vi "LVDimInterface.dis_remove_service.vi"(0 "my_serviceID":i32, 5 "error in (no error)":errorcluster) -> (19 "error out":errorcluster)   [LabVIEW 2015, in "LVDimInterface.lvlib"]
doc: "This routine can be called by the server program when a service stops beeing provided. \nThis routine will inform the Name server and all the clients using this service that it is no longer provided. The service can from then on be provided by another server.\n\nRemark: Please use a \"remove command' for removing command services\n\nHistory: 16-DEC-2005, Dietrich Beck\n\nCopyright (C)\nGesellschaft für Schwerionenforschung, GSI\nPlanckstr. 1\n64291 Darmstadt\nGermany\n\nContact: D.Beck@gsi.de \n\nThis program is free software; you can redistribute it and/or modify it under the terms of the \nGNU General Public License as published by the Free Software Foundation; either version 2 of the license, or (at your option) any later version.\n\nThis program is distributed in the hope that it will be useful, but WITHOUT ANY WARRANTY; without even the implied warranty of MERCHANTABILITY or FITNESS FOR A PARTICULAR PURPOSE. See the GNU General License for more details (http://www.gnu.org).\n\nGesellschaft für Schwerionenforschung, GSI\nPlanckstr. 1, 64291 Darmstadt, Germany\nFor all questions and ideas contact D. Beck.\nLast update: 16-DEC-2005"
uses:
  LVDimInterface.lvlib
  bin/libDimWrapper.dll
  bin/libDimWrapper.so
  bin/libDimWrapperSPL.dll
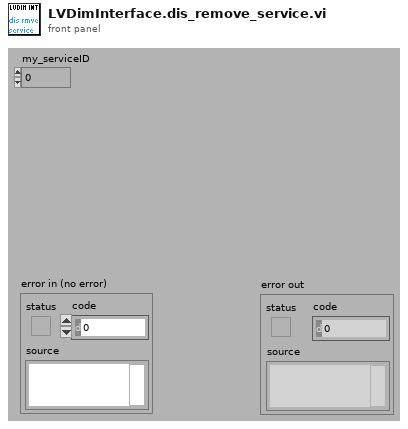
[diagram p1: front panel]
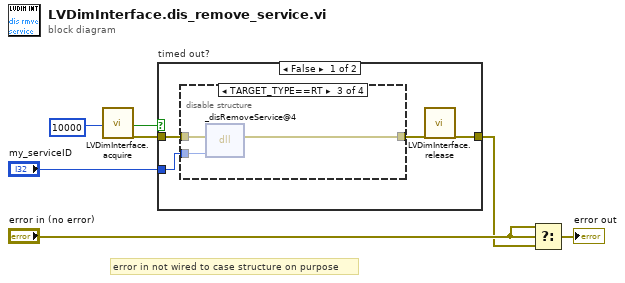
[diagram p0: block diagram]
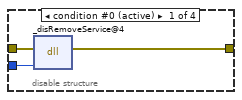
[diagram p2: hidden frame]
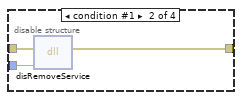
[diagram p3: hidden frame]
diagram:
  # "error in not wired to case structure on purpose"
  n1 = call "LVDimInterface.acquire.vi"("ms timeout (10000)"=10000 ("ms timeout (-1)")) -> ("timed out"=w4:bool, "error out"=w3:errorcluster)  [unwired: 17 in]
  n2 = case "timed out?" shown="False" w4 {
    tunnel: "my_serviceID" -> [w11 _]
    tunnel: w3 -> [w10 w22]
    tunnel: [w8 w22] -> w1
    frame False {
      n3 = disable-structure "Conditional Disable Structure" shown="TARGET_TYPE==RT" {
        disable-tunnel: w11 -> [w14 w17 w20 _]
        disable-tunnel: w10 -> [w13 w16 w19 w21]
        disable-tunnel: [w12 w15 w18 w21] -> w9
        frame condition #0 (active) {
          n4 = dll-call lib="D:/Git/CSPP/Packages/DimLVEvent/bin/libDimWrapper.dll" fn="_disRemoveService@4" label="disRemoveService"(error in=w13, "my_serviceID"=w14) -> (error out=w12:errorcluster)  [unwired: 4 in, 1 out]
        }
        frame condition #1 {
          n5 = dll-call lib="D:/Git/CS-framework/CSlibraries/DimLVEvent/bin/libDimWrapper.so" fn="disRemoveService"(error in=w16, "my_serviceID"=w17) -> (error out=w15:errorcluster)  [unwired: 4 in, 1 out]
        }
        frame condition #2 {
          n6 = dll-call lib="D:/Git/CS-framework/CSlibraries/DimLVEvent/bin/libDimWrapperSPL.dll" fn="_disRemoveService@4" label="libDimWrapper.so:disRemoveService"(error in=w19, "my_serviceID"=w20) -> (error out=w18:errorcluster)  [unwired: 4 in, 1 out]
        }
        frame condition #3 {
        }
      }
      n7 = call "LVDimInterface.release.vi"("error in (no error)"=w9) -> ("error out"=w8:errorcluster)  [unwired: 18 in]
    }
    frame True {
    }
  }
  n8 = Select(t="error in (no error)", s="error in (no error)", f=w1) -> (s? t:f=→"error out":errorcluster)
